vi "GetMaterialPropertiesInConfigDict.vi"(8 "error in (no error)":errorcluster, 10 "MaterialName":string="Material ", 11 "TopLevel in":refnum<class "TopLevel.lvclass">) -> (0 "error out":errorcluster, 2 "Cluster":T1, 3 "TopLevel out":refnum<class "TopLevel.lvclass">)   [LabVIEW 2022 SP3, in "TopLevel.lvclass"]
uses:
  TopLevel.lvclass
  Common/Controls/DLP_MaterialToHeadMapping--Cluster.ctl
  DLP2/DataTypes/DLP2_PrinterMaterialProperties.ctl
  Typedefs/InkIdleNodeConfigXML--Cluster.ctl
  Typedefs/InkProcessNodeConfigXML--Cluster.ctl
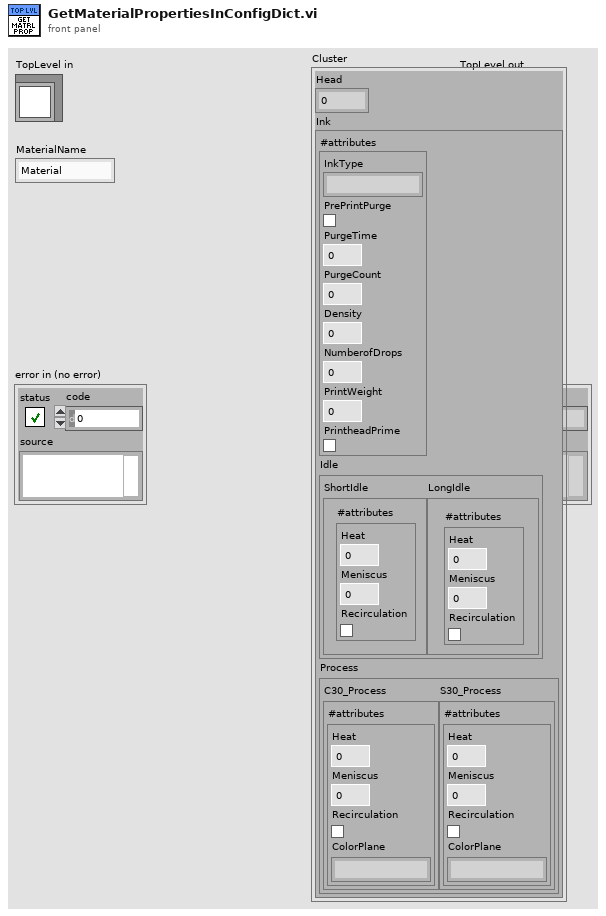
[diagram p1: front panel]
types:
  T1 = typedef "DLP_MaterialToHeadMapping--Cluster.ctl" = cluster{"Head":u8, "Ink":T2}
  T2 = typedef "DLP2_PrinterMaterialProperties.ctl" = cluster{"#attributes":cluster{"InkType":string, "PrePrintPurge":bool, "PurgeTime":dbl, "PurgeCount":i32, "Density":dbl, "NumberofDrops":i32, "PrintWeight":dbl, "PrintheadPrime":bool}, "Idle":T3, "Process":T4}
  T3 = typedef "InkIdleNodeConfigXML--Cluster.ctl" = cluster{"ShortIdle":cluster{"#attributes":cluster{"Heat":dbl, "Meniscus":dbl, "Recirculation":bool}}, "LongIdle":cluster{"#attributes":cluster{"Heat":dbl, "Meniscus":dbl, "Recirculation":bool}}}
  T4 = typedef "InkProcessNodeConfigXML--Cluster.ctl" = cluster{"C30_Process":cluster{"#attributes":cluster{"Heat":dbl, "Meniscus":dbl, "Recirculation":bool, "ColorPlane":string}}, "S30_Process":cluster{"#attributes":cluster{"Heat":dbl, "Meniscus":dbl, "Recirculation":bool, "ColorPlane":string}}}
  T5 = typedef "TD Dynamic CVT DVR--ref.ctl" = refnum<data-value>
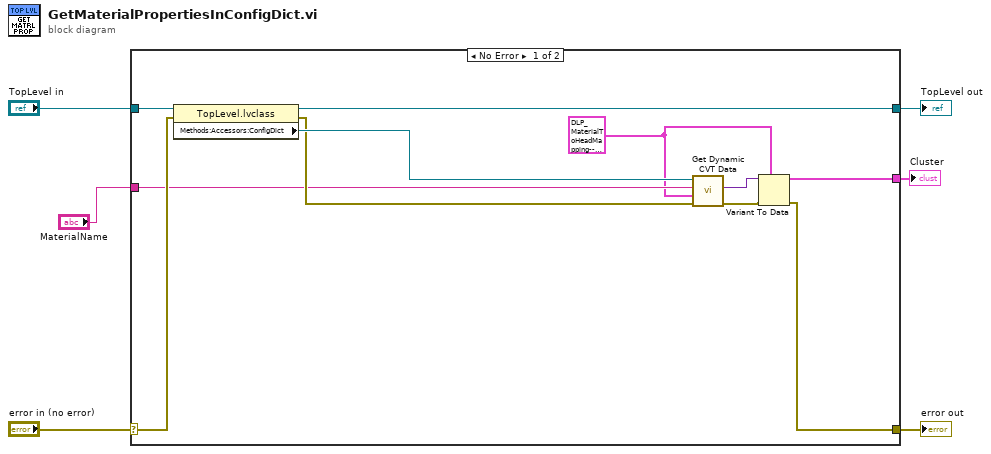
[diagram p0: block diagram]
diagram:
  n1 = case shown="No Error" "error in (no error)" {
    selector: "error in (no error)" -> [w13 w19]
    tunnel: [w10 w19] -> w5
    tunnel: [w15 w18] -> w3
    tunnel: "TopLevel in" -> [w14 w18]
    tunnel: [w9 _] -> w1
    tunnel: "MaterialName" -> [w8 _]
    frame No Error {
      w7 = T1 {"Head"=0, "Ink"={"#attributes"={"InkType"="", "PrePrintPurge"=FALSE, "PurgeTime"=0.0, "PurgeCount"=0, "Density"=0.0, "NumberofDrops"=0, "PrintWeight"=0.0, "PrintheadPrime"=FALSE}, "Idle"={"ShortIdle"={"#attributes"={"Heat"=0.0, "Meniscus"=0.0, "Recirculation"=FALSE}}, "LongIdle"={"#attributes"={"Heat"=0.0, "Meniscus"=0.0, "Recirculation"=FALSE}}}, "Process"={"C30_Process"={"#attributes"={"Heat"=0.0, "Meniscus"=0.0, "Recirculation"=FALSE, "ColorPlane"=""}}, "S30_Process"={"#attributes"={"Heat"=0.0, "Meniscus"=0.0, "Recirculation"=FALSE, "ColorPlane"=""}}}}}
      n2 = property class="TopLevel.lvclass"(reference=w14, error in=w13) -> (reference out=w15:refnum<class "TopLevel.lvclass">, error out=w16:errorcluster, "Methods:Accessors:ConfigDict"=w17:T5)
      n3 = call <vilib>:"Get Dynamic CVT Data.vi"("error in (no error)"=w16, "default value (empty variant)"=w7, "DataName"=w8, "dCVT DVR"=w17) -> ("error out"=w11:errorcluster, "value"=w12:variant)  [unwired: 4 in, 2 out]
      n4 = Variant To Data(error in=w11, type=w7, Variant=w12) -> (data=w9:T1, error out=w10:errorcluster)
    }
    frame Error {
    }
  }
  "error out" <- w5
  "TopLevel out" <- w3
  "Cluster" <- w1
